vi "Ipv.vi"(1 "Gn":dbl, 2 "G":dbl, 3 "Tn":dbl, 4 "T":dbl, 5 "KI":dbl, 6 "Ipvn":dbl) -> (0 "Ipv":dbl)   [LabVIEW 2016]
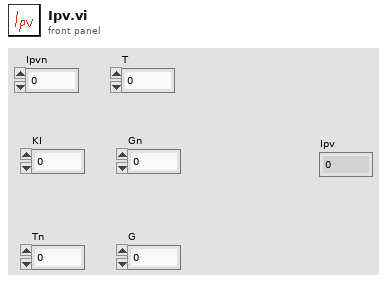
[diagram p1: front panel]
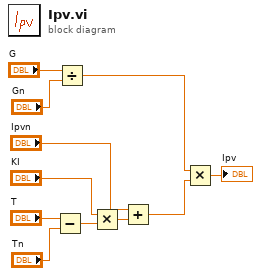
[diagram p0: block diagram]
diagram:
  n1 = Subtract(x="T", y="Tn") -> (x-y=w7:dbl)
  n2 = Divide(x="G", y="Gn") -> (x/y=w1:dbl)
  n3 = Multiply(x="KI", y=w7) -> (x*y=w5:dbl)
  n4 = Add(x="Ipvn", y=w5) -> (x+y=w2:dbl)
  n5 = Multiply(x=w1, y=w2) -> (x*y=→"Ipv":dbl)
